vi "XaxisTime.vi"(5 "Start Time":dbl format="%#_6f", 7 "Stop Time":dbl format="%#_6f", 9 "Points":dbl) -> (8 "X-Axis":dbl[](array[numeric]) format="%#_6f")   [LabVIEW 2018]
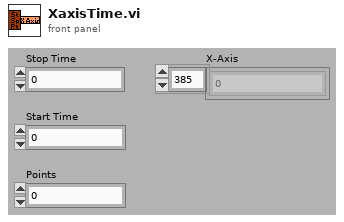
[diagram p1: front panel]
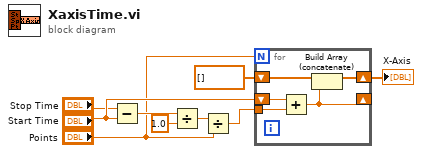
[diagram p0: block diagram]
diagram:
  n1 = Subtract(x="Stop Time", y="Start Time") -> (x-y=w3:dbl)
  n2 = Divide(x=w3, y=1.0) -> (x/y=w4:dbl)
  n3 = Divide(x=w4, y="Points") -> (x/y=w1:dbl)
  n4 = for {
    N: "Points" -> [_]
    tunnel: w1 -> [w14]
    shift-right: [w11] -> w6
    shift-left: dbl[] [] -> [w12]
    shift-right: [w10] -> _
    shift-left: "Start Time" -> [w13]
    n5 = Add(x=w13, y=w14) -> (x+y=w10:dbl)
    n6 = Build Array (concatenate)(w12, w10) -> (w11:dbl[])
  }
  "X-Axis" <- w6
